vi "reading midi file.vi"() -> ()   [LabVIEW 2020]
panel:
  out "HD1-5x":T1
  out "HD1z":string
  out "HD2-5z":T2
  out "Rest of file that contains core file contents":u8[](array[numeric])
  out "HD5a":i16
  out "HD4a":i16
  out "HD3a":i16
  out "HD2a":i32
  out "HD1a":string
  out "HD5b":i16
  out "HD4b":i16
  out "HD3b":i16
  out "HD2b":i32
  out "HD1b":string
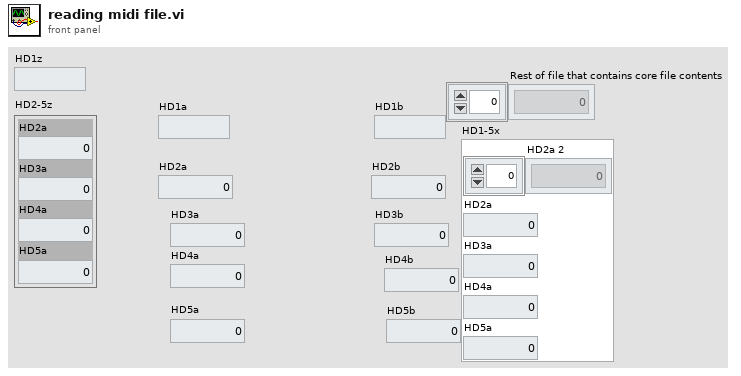
[diagram p1: front panel]
types:
  T1 = cluster{"HD2a 2":u8[], "HD2a":i32, "HD3a":i16, "HD4a":i16, "HD5a":i16}
  T2 = cluster{"HD2a":i32, "HD3a":i16, "HD4a":i16, "HD5a":i16}
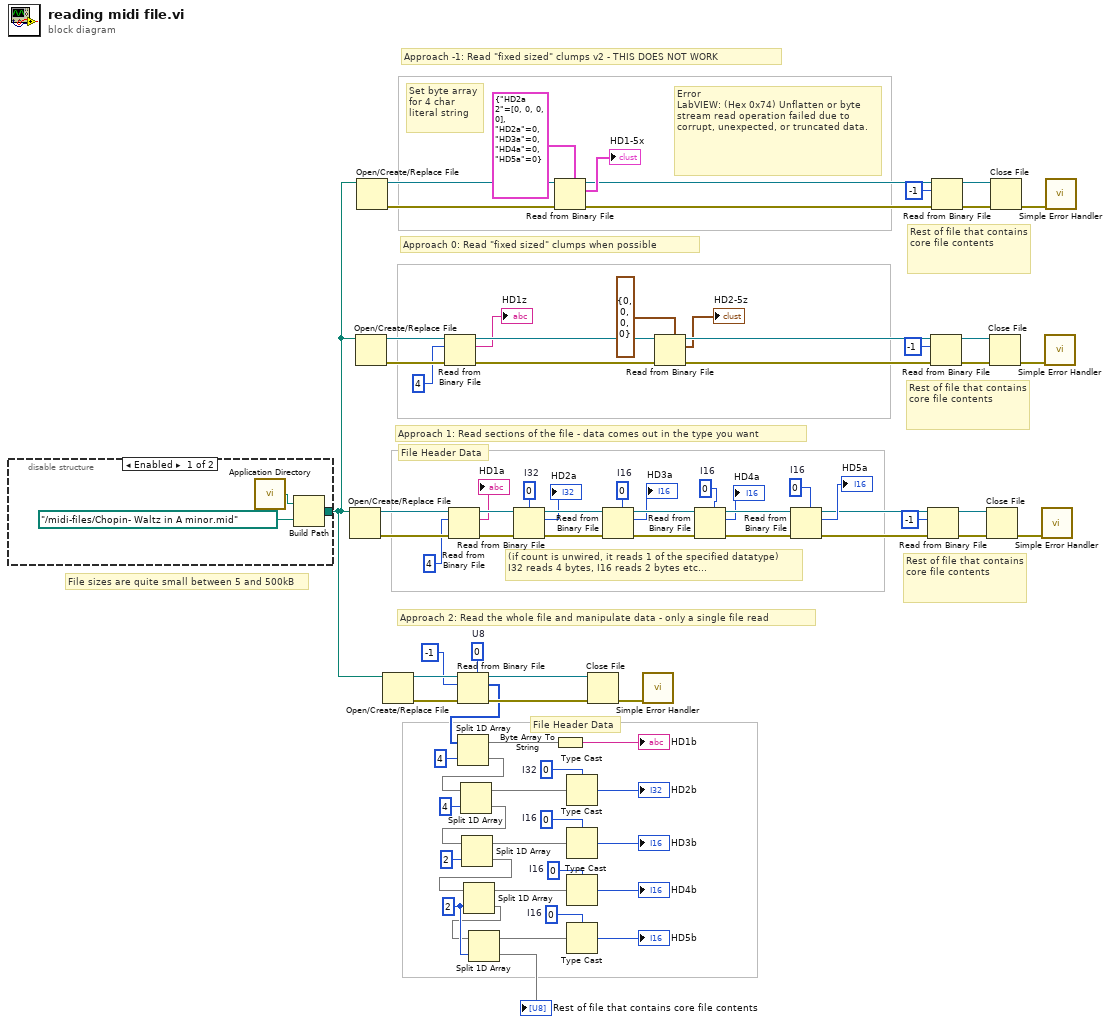
[diagram p0: block diagram]
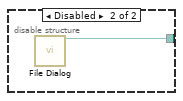
[diagram p2: hidden frame]
diagram:
  w36 = i16 0  # I16
  w35 = i16 0  # I16
  w38 = i16 0  # I16
  w40 = 0  # I32
  w46 = i16 0  # I16
  w49 = i16 0  # I16
  w53 = i16 0  # I16
  w57 = 0  # I32
  w45 = 2 ("index")
  w67 = u8 0  # U8
  # "Error \nLabVIEW: (Hex 0x74) Unflatten or byte stream read operation failed due to corrupt, unexpected, or truncated data."
  # "Set byte array for 4 char literal string"
  # "Approach -1: Read \"fixed sized\" clumps v2 - THIS DOES NOT WORK"
  # "Rest of file that contains core file contents"
  # "Approach 0: Read \"fixed sized\" clumps when possible"
  # "Rest of file that contains core file contents"
  # "Approach 2: Read the whole file and manipulate data - only a single file read"
  # "(if count is unwired, it reads 1 of the specified datatype)\nI32 reads 4 bytes, I16 reads 2 bytes etc..."
  # "Rest of file that contains core file contents"
  # "File sizes are quite small between 5 and 500kB"
  # "Approach 1: Read sections of the file - data comes out in the type you want"
  # "File Header Data"
  # "File Header Data"
  n1 = disable-structure shown="Enabled" {
    disable-tunnel: [w83 w86] -> w7
    frame Enabled {
      n2 = call <vilib>:"Application Directory.vi"() -> ("Application Directory"=w85:path)
      n3 = Build Path(base path=w85, name or relative path=path "../midi-files/Chopin- Waltz in A minor.mid") -> (appended path=w83:path)
    }
    frame Disabled {
      n4 = call "File Dialog"() -> ("selected path"=w86:path)  [unwired: 12 in, 3 out]
    }
  }
  n5 = Open/Create/Replace File(file path (use dialog)=w7) -> (refnum out=w82:refnum<file>, error out=w81:errorcluster)  [unwired: 5 in, 1 out]
  n6 = Open/Create/Replace File(file path (use dialog)=w7) -> (refnum out=w18:refnum<file>, error out=w15:errorcluster)  [unwired: 5 in, 1 out]
  n7 = Open/Create/Replace File(file path (use dialog)=w7) -> (refnum out=w5:refnum<file>, error out=w4:errorcluster)  [unwired: 5 in, 1 out]
  n8 = Open/Create/Replace File(file path (use dialog)=w7) -> (refnum out=w70:refnum<file>, error out=w71:errorcluster)  [unwired: 5 in, 1 out]
  n9 = Read from Binary File(8:w15, 10:4 ("count (1)"), 11:w18) -> (0:w16:errorcluster, 2:→"HD1z":string, 3:w17:refnum<file>)  [unwired: 3 in, 1 out]
  n10 = Read from Binary File(8:w81, 10:4 ("count (1)"), 11:w82) -> (0:w80:errorcluster, 2:→"HD1a":string, 3:w78:refnum<file>)  [unwired: 3 in, 1 out]
  n11 = Read from Binary File(5:w67, 8:w71, 10:-1 ("count (1)"), 11:w70) -> (0:w65:errorcluster, 2:w1:u8[], 3:w66:refnum<file>)  [unwired: 2 in, 1 out]
  n12 = Split 1D Array(array=w1, index=4) -> (first subarray=w55:u8[], second subarray=w61:u8[])
  n13 = Split 1D Array(array=w61, index=4) -> (first subarray=w54:u8[], second subarray=w59:u8[])
  n14 = Split 1D Array(array=w59, index=2) -> (first subarray=w52:u8[], second subarray=w58:u8[])
  n15 = Split 1D Array(array=w58, index=w45) -> (first subarray=w48:u8[], second subarray=w44:u8[])
  n16 = Split 1D Array(array=w44, index=w45) -> (first subarray=w43:u8[], second subarray=→"Rest of file that contains core file contents":u8[])
  n17 = Read from Binary File(5:w40, 8:w80, 11:w78) -> (0:w72:errorcluster, 2:→"HD2a":i32, 3:w75:refnum<file>)  [unwired: 3 in, 1 out]
  n18 = Read from Binary File(5:T1 {"HD2a 2"=[0, 0, 0, 0], "HD2a"=0, "HD3a"=0, "HD4a"=0, "HD5a"=0} ("Cluster"), 8:w4, 11:w5) -> (0:w3:errorcluster, 2:→"HD1-5x":T1, 3:w2:refnum<file>)  [unwired: 3 in, 1 out]
  n19 = Byte Array To String(unsigned byte array=w55) -> (string=→"HD1b":string)
  n20 = Type Cast(type=w57, x=w54) -> (*(type *) &x=→"HD2b":i32)
  n21 = Type Cast(type=w53, x=w52) -> (*(type *) &x=→"HD3b":i16)
  n22 = Type Cast(type=w49, x=w48) -> (*(type *) &x=→"HD4b":i16)
  n23 = Type Cast(type=w46, x=w43) -> (*(type *) &x=→"HD5b":i16)
  n24 = Close File(refnum=w66, error in=w65) -> (error out=w69:errorcluster)  [unwired: 1 out]
  n25 = Read from Binary File(5:w38, 8:w72, 11:w75) -> (0:w74:errorcluster, 2:→"HD3a":i16, 3:w77:refnum<file>)  [unwired: 3 in, 1 out]
  n26 = call <vilib>:"Simple Error Handler.vi"("error in (no error)"=w69) -> ()  [unwired: 4 in, 5 out]
  n27 = Read from Binary File(5:T2 {"HD2a"=0, "HD3a"=0, "HD4a"=0, "HD5a"=0} ("Cluster"), 8:w16, 11:w17) -> (0:w19:errorcluster, 2:→"HD2-5z":T2, 3:w22:refnum<file>)  [unwired: 3 in, 1 out]
  n28 = Read from Binary File(5:w35, 8:w74, 11:w77) -> (0:w73:errorcluster, 2:→"HD4a":i16, 3:w76:refnum<file>)  [unwired: 3 in, 1 out]
  n29 = Read from Binary File(5:w36, 8:w73, 11:w76) -> (0:w28:errorcluster, 2:→"HD5a":i16, 3:w31:refnum<file>)  [unwired: 3 in, 1 out]
  n30 = Read from Binary File(8:w28, 10:-1 ("count (1)"), 11:w31) -> (0:w29:errorcluster, 3:w30:refnum<file>)  [unwired: 3 in, 2 out]
  n31 = Read from Binary File(8:w19, 10:-1 ("count (1)"), 11:w22) -> (0:w25:errorcluster, 3:w24:refnum<file>)  [unwired: 3 in, 2 out]
  n32 = Read from Binary File(8:w3, 10:-1 ("count (1)"), 11:w2) -> (0:w9:errorcluster, 3:w10:refnum<file>)  [unwired: 3 in, 2 out]
  n33 = Close File(refnum=w30, error in=w29) -> (error out=w79:errorcluster)  [unwired: 1 out]
  n34 = Close File(refnum=w24, error in=w25) -> (error out=w23:errorcluster)  [unwired: 1 out]
  n35 = Close File(refnum=w10, error in=w9) -> (error out=w11:errorcluster)  [unwired: 1 out]
  n36 = call <vilib>:"Simple Error Handler.vi"("error in (no error)"=w79) -> ()  [unwired: 4 in, 5 out]
  n37 = call <vilib>:"Simple Error Handler.vi"("error in (no error)"=w23) -> ()  [unwired: 4 in, 5 out]
  n38 = call <vilib>:"Simple Error Handler.vi"("error in (no error)"=w11) -> ()  [unwired: 4 in, 5 out]
